vi "2-1mux_int.vi"(6 "Select":bool, 9 "Input2":dbl, 11 "Input1":dbl) -> (2 "Output":dbl)   [LabVIEW 2011]
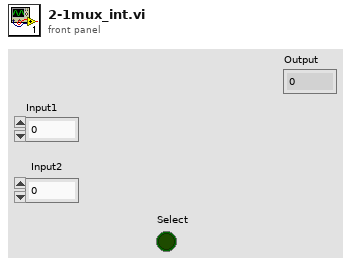
[diagram p1: front panel]
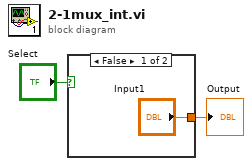
[diagram p0: block diagram]
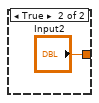
[diagram p2: hidden frame]
diagram:
  n1 = case shown="False" "Select" {
    tunnel: ["Input1" "Input2"] -> w2
    frame False {
    }
    frame True {
    }
  }
  "Output" <- w2
